vi "Test RND Integer.vi"() -> ()   [LabVIEW 2015]
uses:
  TSP Library/TSP Library.lvlib
  <vilib>/Analysis/NI_AALBase.lvlib
panel:
  in  "Min":i32=1
  in  "Max":i32=9
  out "Histogram Graph":T1(graph)
  in  "intervals":i32=33
  out "min value":i32
  out "max value":i32
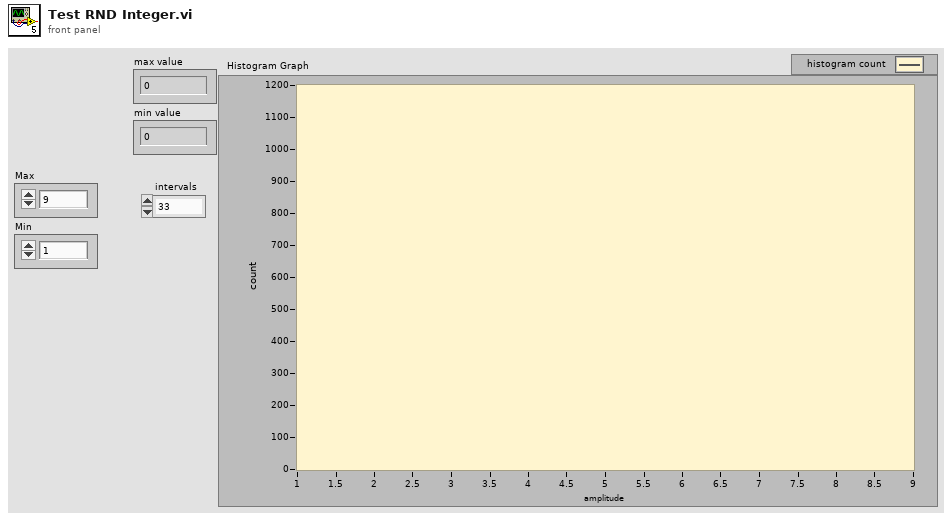
[diagram p1: front panel]
types:
  T1 = cluster{"X Values":dbl[], "Histogram: h(x)":i32[]}
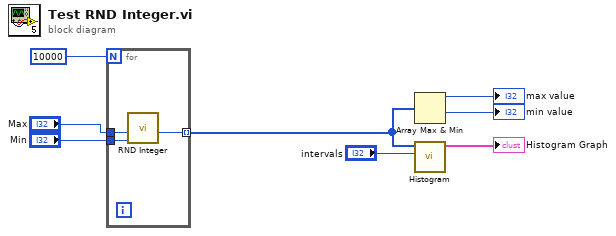
[diagram p0: block diagram]
diagram:
  n1 = for {
    N: 10000 -> [_]
    tunnel: [w11] -> w5 mode=indexing
    tunnel: "Min" -> [w10]
    tunnel: "Max" -> [w9]
    n2 = call "RND Integer.vi"("Min"=w10, "Max"=w9) -> ("RND Integer"=w11:i32)  [unwired: 9 in]
  }
  n3 = Array Max & Min(array=w5) -> (max value=→"max value":i32, min value=→"min value":i32)  [unwired: 2 out]
  n4 = call <vilib>:"Histogram.vi"("intervals"="intervals", "X"=w5) -> ("Histogram Graph"=→"Histogram Graph":T1)  [unwired: 6 in, 3 out]
